vi "DetectDev.vi"(1 "IP.":string caption="IP地址") -> (0 "Fail":bool)   [LabVIEW 2012]
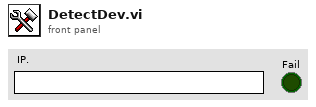
[diagram p1: front panel]
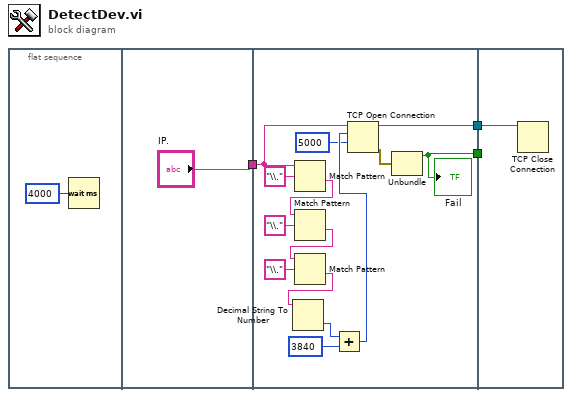
[diagram p0: block diagram]
diagram:
  n1 = flat-sequence {
    tunnel: ["IP."] -> w3
    tunnel: w3 -> [w14]
    tunnel: [w8] -> w2
    tunnel: [w7] -> w1
    tunnel: w2 -> [w20]
    tunnel: w1 -> [_]
    frame #0 {
      n2 = Wait (ms)(milliseconds to wait=u32 4000 ("等待时间（毫秒）")) -> ()  [unwired: 1 out]
    }
    frame #1 {
    }
    frame #2 {
      n3 = Match Pattern(string=w14, regular expression="\\." ("正则表达式")) -> (after substring=w16:string)  [unwired: 1 in, 3 out]
      n4 = Match Pattern(string=w16, regular expression="\\." ("正则表达式")) -> (after substring=w15:string)  [unwired: 1 in, 3 out]
      n5 = Match Pattern(string=w15, regular expression="\\." ("正则表达式")) -> (after substring=w13:string)  [unwired: 1 in, 3 out]
      n6 = Decimal String To Number(string=w13) -> (number=w12:i32)  [unwired: 2 in, 1 out]
      n7 = Add(x=w12, y=3840) -> (x+y=w10:i32)
      n8 = TCP Open Connection(address=w14, remote port or service name=w10, timeout ms (60000)=5000 ("超时毫秒(60000)")) -> (connection ID=w8:refnum<k5>, error out=w9:errorcluster)  [unwired: 2 in]
      n9 = Unbundle(w9) -> ("status"=w7:bool)  [unwired: 2 out]
      "Fail" <- w7
    }
    frame #3 {
      n10 = TCP Close Connection(connection ID=w20) -> ()  [unwired: 2 in, 2 out]
    }
  }
